vi "niRFUtil FTW Apply Window (real wfm).vi"(3 "Window":T1=enum."Gaussian", 5 "Waveform In":T2 {"y" min=0 max=127 format="%.2f"; "dx" format="%^.2e"; "x0" format="%^.2e"}) -> (0 "-ENBW (dB-Hz)":sgl format="%.2f", 1 "Coherent Loss (dB)":sgl format="%.2f", 2 "Waveform Out":T2 {"y" min=0 max=127 format="%.2f"; "dx" format="%^.2e"; "x0" format="%^.2e"})   [LabVIEW 2015, in "niRFUtil.lvlib"]
doc: "(c) Copyright 2006, National Instruments, Inc. This VI may not be duplicated, sold, or distributed without written consent from National Instruments."
uses:
  niRFUtil.lvlib
  Includes/niRFUtil INC Real Waveform.ctl
  Includes/niRFUtil INC Real Array.ctl
  Includes/niRFUtil INC FFT Window.ctl
  <vilib>/Analysis/4window.llb/Hanning Window (DBL).vi
  <vilib>/Analysis/4window.llb/Hamming Window (DBL).vi
  <vilib>/Analysis/4window.llb/Gaussian Window (DBL).vi
  <vilib>/Analysis/4window.llb/Blackman Window (DBL).vi
  <vilib>/Analysis/4window.llb/Blackman-Harris Window (DBL).vi
  <vilib>/Analysis/4window.llb/Kaiser-Bessel Window (DBL).vi
  <vilib>/Analysis/4window.llb/AllCosWindow (DBL).vi
  <vilib>/Analysis/NI_AALPro.lvlib
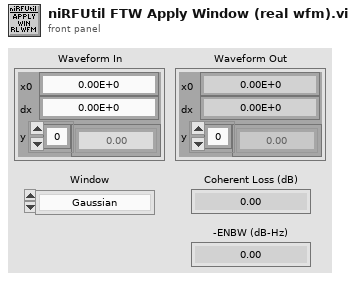
[diagram p1: front panel]
types:
  T1 = typedef "niRFUtil.lvlib/niRFUtil INC FFT Window.ctl" = enum16{"None", "Flat Top", "Hanning", "Hamming", "Gaussian", "Blackman", "Blackman-Harris", "Kaiser-Bessel 70 dB", "Kaiser-Bessel 90 dB", "Kaiser-Bessel 110 dB"}
  T2 = typedef "niRFUtil.lvlib/niRFUtil INC Real Waveform.ctl" = cluster{"x0":dbl, "dx":dbl, "y":T3}
  T3 = typedef "niRFUtil.lvlib/niRFUtil INC Real Array.ctl" = sgl[]
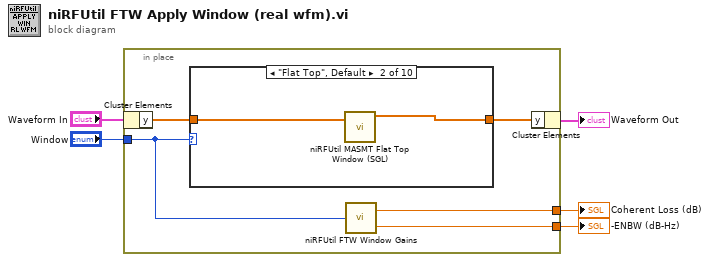
[diagram p0: block diagram]
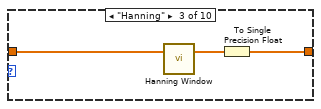
[diagram p3: hidden frame]
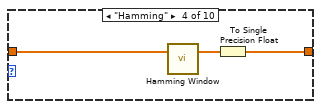
[diagram p4: hidden frame]
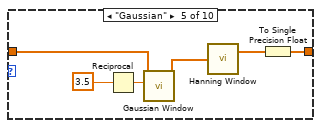
[diagram p5: hidden frame]
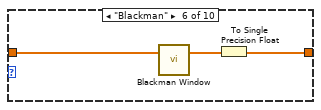
[diagram p6: hidden frame]
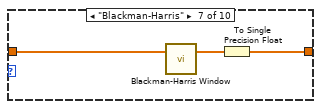
[diagram p7: hidden frame]
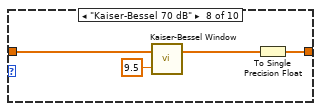
[diagram p8: hidden frame]
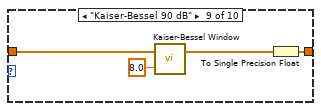
[diagram p9: hidden frame]
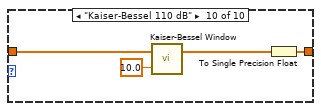
[diagram p10: hidden frame]
diagram:
  n1 = in-place {
    in-place-border: "Window" -> [w10]
    in-place-border: [w9] -> w4
    in-place-border: [w8] -> w3
    n2 = in-place-cluster #1("Waveform In") -> ("y"=w7:T3)
    n3 = case shown="\"Flat Top\", Default" w10 {
      tunnel: w7 -> [w11 w13 w16 w19 w25 w28 w31 w35 w39 w43]
      tunnel: [w11 w12 w14 w17 w20 w26 w29 w33 w37 w41] -> w6
      frame "None" {
      }
      frame "Flat Top", Default {
        n4 = call "niRFUtil MASMT Flat Top Window (SGL).vi"("X"=w13) -> ("Windowed X"=w12:sgl[])  [unwired: 9 in, 1 out]
      }
      frame "Hanning" {
        n5 = call-poly <vilib>:"Hanning Window.vi"("X"=w16) -> ("Windowed X"=w15:dbl[])  [unwired: 1 out]
        n6 = To Single Precision Float(number=w15) -> (single precision float=w14:sgl[])
      }
      frame "Hamming" {
        n7 = call-poly <vilib>:"Hamming Window.vi"("X"=w19) -> ("Windowed X"=w18:dbl[])  [unwired: 1 out]
        n8 = To Single Precision Float(number=w18) -> (single precision float=w17:sgl[])
      }
      frame "Gaussian" {
        n9 = Reciprocal(x=3.5 ("standard deviation")) -> (1/x=w23:dbl)
        n10 = call-poly <vilib>:"Gaussian Window.vi"("standard deviation"=w23, "X"=w25) -> ("Windowed X"=w22:dbl[])  [unwired: 9 out]
        n11 = call-poly <vilib>:"Hanning Window.vi"("X"=w22) -> ("Windowed X"=w21:dbl[])  [unwired: 1 out]
        n12 = To Single Precision Float(number=w21) -> (single precision float=w20:sgl[])
      }
      frame "Blackman" {
        n13 = call-poly <vilib>:"Blackman Window.vi"("X"=w28) -> ("Windowed X"=w27:dbl[])  [unwired: 1 out]
        n14 = To Single Precision Float(number=w27) -> (single precision float=w26:sgl[])
      }
      frame "Blackman-Harris" {
        n15 = call-poly <vilib>:"Blackman-Harris Window.vi"("X"=w31) -> ("Windowed X"=w30:dbl[])  [unwired: 1 out]
        n16 = To Single Precision Float(number=w30) -> (single precision float=w29:sgl[])
      }
      frame "Kaiser-Bessel 70 dB" {
        n17 = call-poly <vilib>:"Kaiser-Bessel Window.vi"("beta"=9.5, "X"=w35) -> ("Windowed X"=w32:dbl[])  [unwired: 1 out]
        n18 = To Single Precision Float(number=w32) -> (single precision float=w33:sgl[])
      }
      frame "Kaiser-Bessel 90 dB" {
        n19 = call-poly <vilib>:"Kaiser-Bessel Window.vi"("beta"=8.0, "X"=w39) -> ("Windowed X"=w36:dbl[])  [unwired: 1 out]
        n20 = To Single Precision Float(number=w36) -> (single precision float=w37:sgl[])
      }
      frame "Kaiser-Bessel 110 dB" {
        n21 = call-poly <vilib>:"Kaiser-Bessel Window.vi"("beta"=10.0, "X"=w43) -> ("Windowed X"=w40:dbl[])  [unwired: 1 out]
        n22 = To Single Precision Float(number=w40) -> (single precision float=w41:sgl[])
      }
    }
    n23 = call "niRFUtil FTW Window Gains.vi"("Window"=w10) -> ("-ENBW (dB-Hz)"=w8:sgl, "Coherent Loss (dB)"=w9:sgl)  [unwired: 2 in]
    n24 = in-place-cluster #1("y"=w6) -> (→"Waveform Out":T2)
  }
  "-ENBW (dB-Hz)" <- w3
  "Coherent Loss (dB)" <- w4
